vi "ReadWritePython.vi"(6 "Reply length":i32=-1, 7 "Send as 1 block?":bool, 8 "error in":errorcluster, 9 "Console In":string, 10 "Write":string, 11 "VISA in":refnum<visa-resource-name>) -> (0 "error out":errorcluster, 1 "Console Out":string, 2 "Update?":bool, 3 "VISA out":refnum<visa-resource-name>, 4 "Not Done?":bool, 5 "read buffer":string)   [LabVIEW 2016]
panel:
  out "Bytes at Port":u32
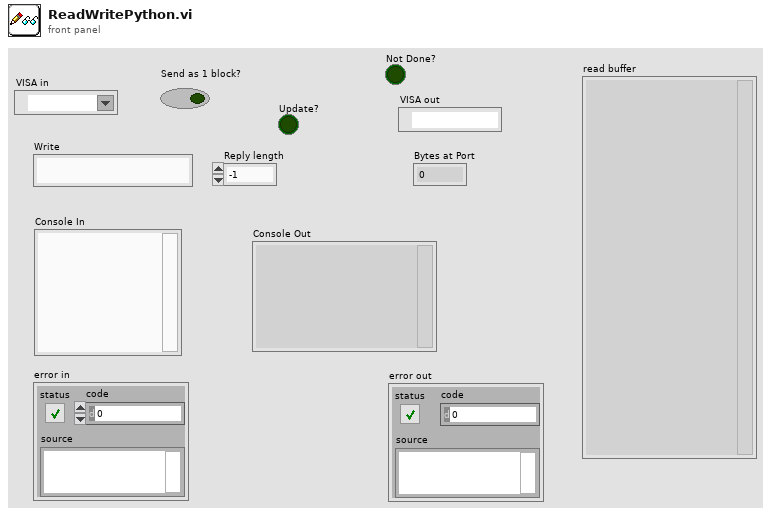
[diagram p1: front panel]
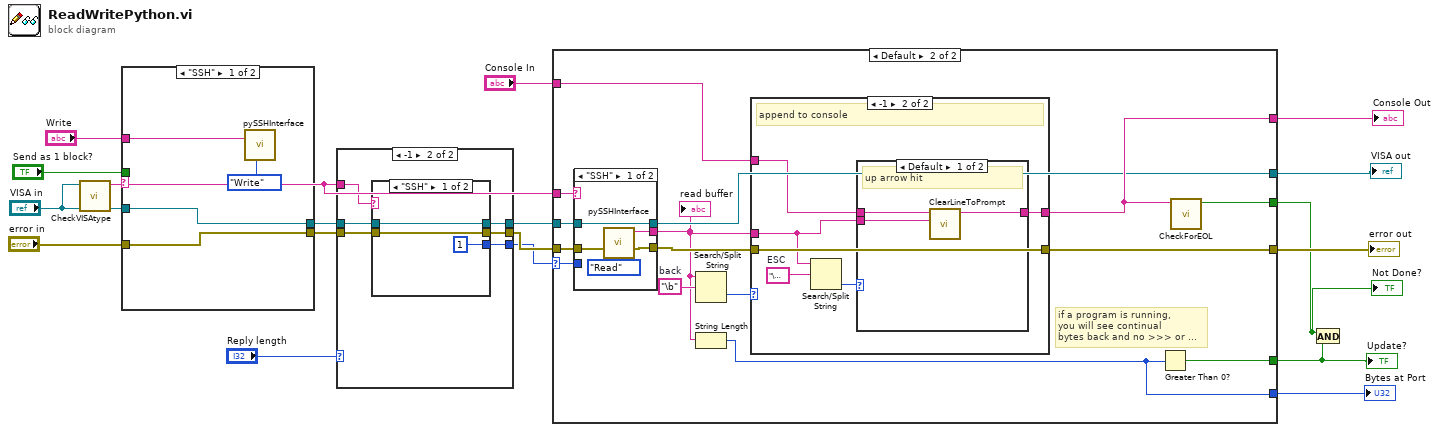
[diagram p0: block diagram]
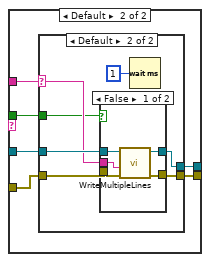
[diagram p2: hidden frame]
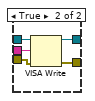
[diagram p4: hidden frame]
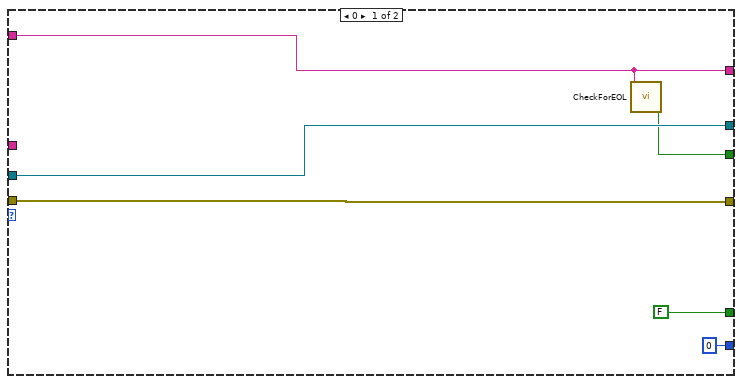
[diagram p5: hidden frame]
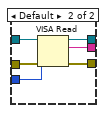
[diagram p6: hidden frame]
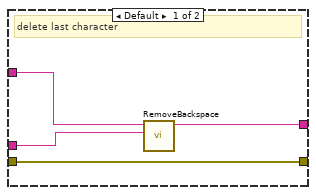
[diagram p7: hidden frame]
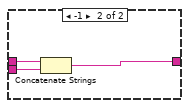
[diagram p8: hidden frame]
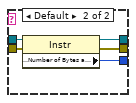
[diagram p10: hidden frame]
diagram:
  n1 = call "CheckVISAtype.vi"("VISA Refnum in"="VISA in") -> ("data string"=w2:string)  [unwired: 9 in, 1 out]
  n2 = case shown="\"SSH\"" w2 {
    tunnel: "Write" -> [w21 w28]
    tunnel: "error in" -> [w19 w27]
    tunnel: "VISA in" -> [w20 w26]
    tunnel: [w19 w25] -> w11
    tunnel: [w20 w24] -> w10
    tunnel: "Send as 1 block?" -> [_ w23]
    frame "SSH" {
      n3 = call "pySSHInterface.vi"("Task"=enum16{"Init", "Read", "Write", "Close"}."Write", "String to write"=w21) -> ()  [unwired: 9 in, 1 out]
    }
    frame Default {
      n4 = case shown="Default" w28 {
        selector: w28 -> [_ w33]
        tunnel: w26 -> [w30 w36]
        tunnel: w27 -> [w29 w35]
        tunnel: [w30 w32] -> w24
        tunnel: [w29 w34] -> w25
        tunnel: w23 -> [_ w31]
        frame "" {
        }
        frame Default {
          n5 = case shown="False" w31 {
            tunnel: w36 -> [w42 w47]
            tunnel: w35 -> [w41 w45]
            tunnel: [w40 w43] -> w34
            tunnel: w33 -> [w39 w46]
            tunnel: [w38 w44] -> w32
            frame False {
              n6 = call "WriteMultipleLines.vi"("error in"=w41, "Text to write"=w39, "VISA resource name"=w42) -> ("error out"=w40:errorcluster, "VISA Refnum out"=w38:refnum<visa-resource-name>)  [unwired: 7 in]
            }
            frame True {
              n7 = VISA Write(VISA resource name=w47, write buffer=w46, error in (no error)=w45) -> (VISA resource name out=w44:refnum<visa-resource-name>, error out=w43:errorcluster)  [unwired: 1 out]
            }
          }
          n8 = Wait (ms)(milliseconds to wait=u32 1) -> ()  [unwired: 1 out]
        }
      }
    }
  }
  n9 = case shown="-1" "Reply length" {
    selector: "Reply length" -> [w48 _]
    tunnel: [w50 w56] -> w9
    tunnel: [w48 w55] -> w4
    tunnel: w10 -> [w50 w54]
    tunnel: w11 -> [w49 w53]
    tunnel: [w49 w52] -> w8
    tunnel: w2 -> [_ w51]
    frame Default {
    }
    frame -1 {
      n10 = case shown="\"SSH\"" w51 {
        tunnel: [w59 w64] -> w56
        tunnel: [u32 1 ("Bytes at Port") w63] -> w55
        tunnel: w54 -> [w59 w62]
        tunnel: w53 -> [w58 w61]
        tunnel: [w58 w60] -> w52
        frame "SSH" {
        }
        frame Default {
          n11 = property class="Instr"(reference=w62, error in=w61) -> (reference out=w64:refnum<visa-resource-name>, error out=w60:errorcluster, "Serial Settings:Number of Bytes at Serial Port"=w63:u32)
        }
      }
    }
  }
  n12 = case shown="Default" w4 {
    selector: w4 -> [_ w74]
    tunnel: [w66 w85] -> w16
    tunnel: [w69 w84] -> w15
    tunnel: "Console In" -> [w66 w83]
    tunnel: [w70 w82] -> w13
    tunnel: w9 -> [w70 w79]
    tunnel: w8 -> [w69 w78]
    tunnel: [w67 w77] -> w7
    tunnel: [FALSE w76] -> w6
    tunnel: w2 -> [_ w73]
    tunnel: [0 w71] -> w1
    frame 0 {
      n13 = call "CheckForEOL.vi"("String"=w66) -> ("NOT EOL?"=w67:bool)  [unwired: 10 in]
    }
    frame Default {
      w81 = "\b"  # back
      # "if a program is running,\nyou will see continual\nbytes back and no >>> or ..."
      n14 = case shown="\"SSH\"" w73 {
        tunnel: [w89 w95] -> w82
        tunnel: [w86 w94] -> w72
        tunnel: [w88 w93] -> w80
        tunnel: w79 -> [w89 w92]
        tunnel: w78 -> [w88 w91]
        tunnel: w74 -> [_ w90]
        frame "SSH" {
          n15 = call "pySSHInterface.vi"("Task"=enum16{"Init", "Read", "Write", "Close"}."Read") -> ("reply"=w86:string)  [unwired: 10 in]
        }
        frame Default {
          n16 = VISA Read(VISA resource name=w92, byte count=w90, error in (no error)=w91) -> (VISA resource name out=w95:refnum<visa-resource-name>, read buffer=w94:string, error out=w93:errorcluster)  [unwired: 1 out]
        }
      }
      "read buffer" <- w72
      n17 = Search/Split String(string=w72, search string/char (-)=w81) -> (offset of match=w75:i32)  [unwired: 1 in, 2 out]
      n18 = String Length(string=w72) -> (length=w71:i32)
      n19 = case shown="-1" w75 {
        tunnel: w72 -> [w96 w102]
        tunnel: w83 -> [w99 w105]
        tunnel: [w97 w104] -> w85
        tunnel: w80 -> [w98 w103]
        tunnel: [w98 w103] -> w84
        frame Default {
          # "delete last character"
          n20 = call "RemoveBackspace.vi"("read buffer"=w96, "Console In"=w99) -> ("String"=w97:string)  [unwired: 9 in]
        }
        frame -1 {
          w100 = "\u001b"  # ESC
          # "append to console"
          n21 = Search/Split String(string=w102, search string/char (-)=w100) -> (offset of match=w101:i32)  [unwired: 1 in, 2 out]
          n22 = case shown="Default" w101 {
            tunnel: w105 -> [w108 w111]
            tunnel: [w107 w110] -> w104
            tunnel: w102 -> [w106 w109]
            frame Default {
              # "up arrow hit"
              n23 = call "ClearLineToPrompt.vi"("read buffer"=w106, "Console In"=w108) -> ("String"=w107:string)  [unwired: 9 in]
            }
            frame -1 {
              n24 = Concatenate Strings(w111, w109) -> (w110:string)
            }
          }
        }
      }
      n25 = Greater Than 0?(x=w71) -> (x > 0?=w76:bool)
      n26 = call "CheckForEOL.vi"("String"=w85) -> ("NOT EOL?"=w77:bool)  [unwired: 10 in]
    }
  }
  "Not Done?" <- w7
  "Update?" <- w6
  "Bytes at Port" <- w1
  "Console Out" <- w16
  "error out" <- w15
  "VISA out" <- w13
  n27 = And(x=w7, y=w6) -> ()  [unwired: 1 out]
